vi "And.vi"(2 "B":bool, 3 "A":bool) -> (0 "Output":bool)   [LabVIEW 2020, in "Hack.lvlib"]
uses:
  Hack.lvlib
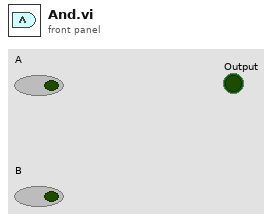
[diagram p1: front panel]
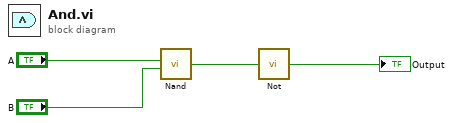
[diagram p0: block diagram]
diagram:
  n1 = call "Nand.vi"("B"="B", "A"="A") -> ("Output"=w2:bool)  [unwired: 2 in]
  n2 = call "Not.vi"("Input"=w2) -> ("Output"=→"Output":bool)
